vi "GlobalDefault.vi"(1 "Write Default":u16, 2 "Write?":bool) -> (0 "Default":u16)   [LabVIEW 2010, in "FTC.lvlib" / "Remote Interface.lvlib"]
uses:
  Remote Interface.lvlib
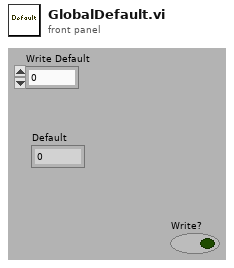
[diagram p1: front panel]
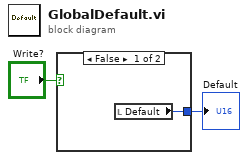
[diagram p0: block diagram]
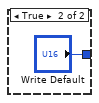
[diagram p2: hidden frame]
diagram:
  n1 = case shown="False" "Write?" {
    tunnel: [w3 "Write Default"] -> w1
    frame False {
      n2 = local read "Default"() -> (w3:u16)
    }
    frame True {
    }
  }
  "Default" <- w1
